vi "SNR.vi"(10 "ROI":T2, 11 "Refnum in":T1) -> (3 "SNR Results":T3)   [LabVIEW 2023]
uses:
  <vilib>/vision/Image Controls.llb/IMAQ Image.ctl
  <vilib>/vision/NI_Vision_Development_Module.lvlib
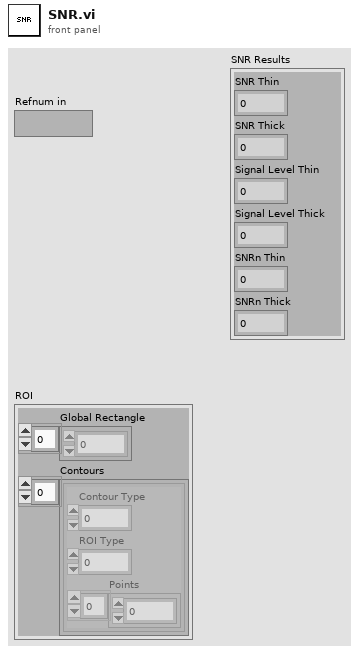
[diagram p1: front panel]
types:
  T1 = typedef "IMAQ Image.ctl" = refnum<image>
  T2 = cluster{"Global Rectangle":i32[], "Contours":cluster{"Contour Type":u32, "ROI Type":u32, "Points":i32[]}[]}
  T3 = cluster{"SNR Thin":sgl, "SNR Thick":sgl, "Signal Level Thin":sgl, "Signal Level Thick":sgl, "SNRn Thin":sgl, "SNRn Thick":sgl}
  T4 = typedef "ROI Descriptor" = cluster{"Global Rectangle":i32[], "Contours":cluster{"ID":enum32{"External", "Internal"}, "Type":u32, "Coordinates":i32[]}[]}
  T5 = cluster{"histogram":u32[], "Minimal Value":sgl, "Maximal Value":sgl, "Starting Value":sgl, "Interval Width":sgl, "Mean Value":sgl, "Standard  Variation":sgl, "Area (pixels)":i32}
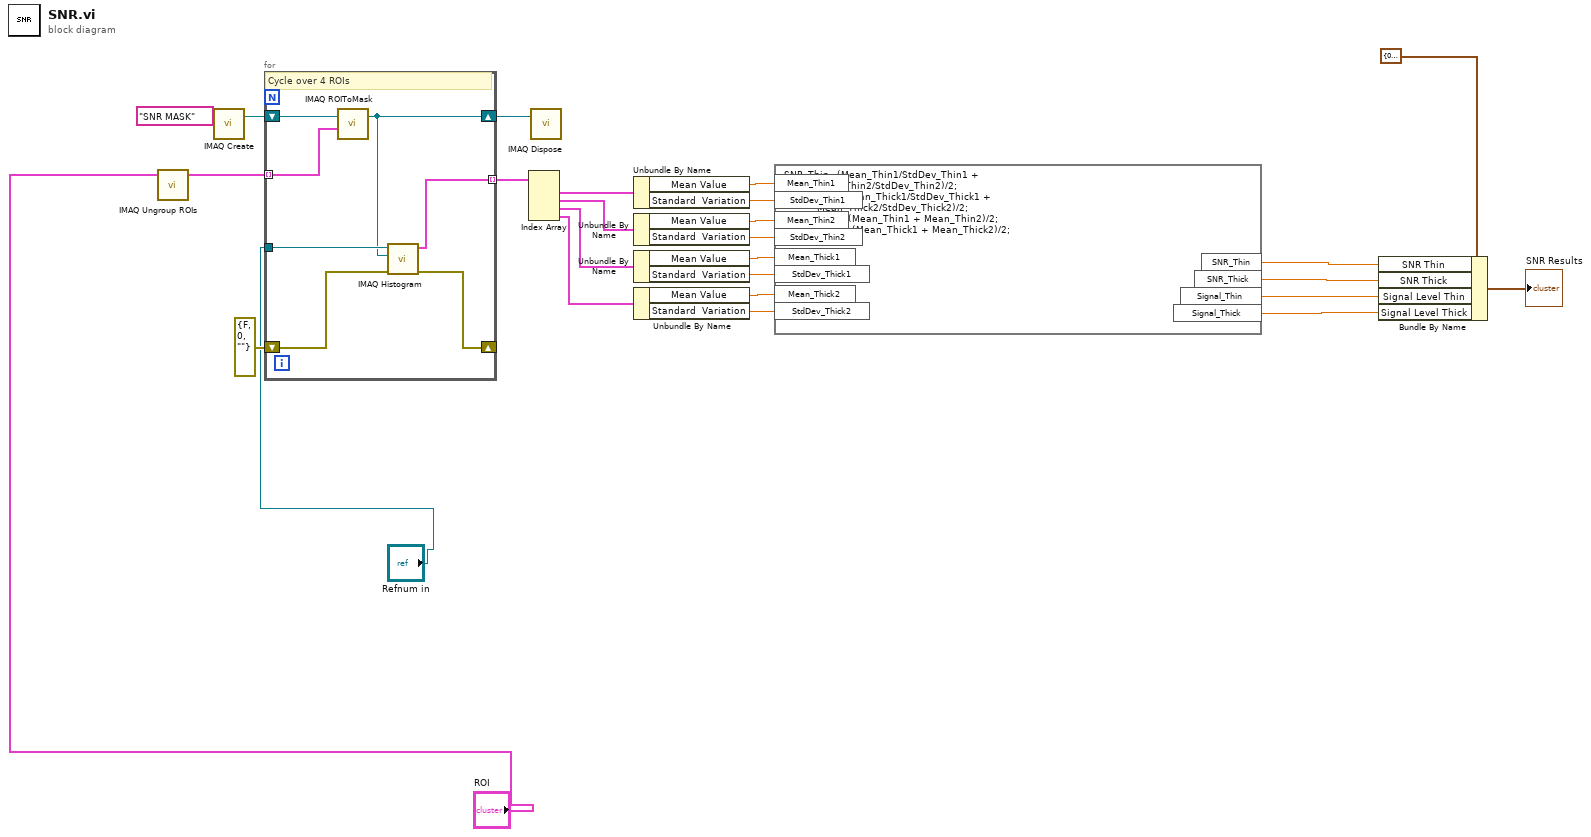
[diagram p0: block diagram]
diagram:
  n1 = call "IMAQ Ungroup ROIs"("ROI Descriptor"="ROI") -> ("ROI Descriptors out"=w3:T4[])  [unwired: 3 in, 1 out]
  n2 = call "IMAQ Create"("Image Name"="SNR MASK") -> ("New Image"=w5:T1)  [unwired: 3 in, 2 out]
  n3 = for {
    tunnel: "Refnum in" -> [w32]
    shift-right: [w28] -> _
    shift-left: errorcluster {"status"=FALSE, "code"=0, "source"=""} ("error out") -> [w31]
    tunnel: w3 -> [w30] mode=indexing
    shift-right: [w29] -> w2
    shift-left: w5 -> [w33]
    tunnel: [w27] -> w22 mode=indexing
    # "Cycle over 4 ROIs"
    n4 = call "IMAQ ROIToMask"("ROI Descriptor"=w30, "Image"=w33) -> ("Image Out"=w29:T1)  [unwired: 3 in, 3 out]
    n5 = call "IMAQ Histogram"("error in (no error)"=w31, "Image Mask"=w29, "Image"=w32) -> ("error out"=w28:errorcluster, "Histogram Report"=w27:T5)  [unwired: 2 in, 5 out]
  }
  n6 = Index Array(array=w22) -> (element #1=w6:T5, element #2=w7:T5, element #3=w8:T5, element #4=w9:T5)  [unwired: 4 in]
  n7 = call "IMAQ Dispose"("Image"=w2) -> ()  [unwired: 2 in, 4 out]
  n8 = Unbundle By Name(w6) -> ("Mean Value"=w10:sgl, "Standard  Variation"=w11:sgl)
  n9 = Unbundle By Name(w7) -> ("Mean Value"=w12:sgl, "Standard  Variation"=w13:sgl)
  n10 = Unbundle By Name(w8) -> ("Mean Value"=w14:sgl, "Standard  Variation"=w15:sgl)
  n11 = Unbundle By Name(w9) -> ("Mean Value"=w16:sgl, "Standard  Variation"=w17:sgl)
  n12 = formula code="SNR_Thin=(Mean_Thin1/StdDev_Thin1 + \n          Mean_Thin2/StdDev_Thin2)/2;\nSNR_Thick=(Mean_Thick1/StdDev_Thick1 + \n           Mean_Thick2/StdDev_Thick2)/2;\nSignal_Thin=(Mean_Thin1 + Mean_Thin2)/2;\nSignal_Thick=(Mean_Thick1 + Mean_Thick2)/2;"("Mean_Thin1"=w10, "Mean_Thin2"=w12, "StdDev_Thin1"=w11, "StdDev_Thin2"=w13, "Mean_Thick1"=w14, "StdDev_Thick1"=w15, "Mean_Thick2"=w16, "StdDev_Thick2"=w17) -> ("SNR_Thin"=w18:dbl, "SNR_Thick"=w19:dbl, "Signal_Thin"=w20:dbl, "Signal_Thick"=w21:dbl)
  n13 = Bundle By Name(cluster=T3 {"SNR Thin"=0.0, "SNR Thick"=0.0, "Signal Level Thin"=0.0, "Signal Level Thick"=0.0, "SNRn Thin"=0.0, "SNRn Thick"=0.0} ("SNR Results"), "SNR Thin"=w18, "SNR Thick"=w19, "Signal Level Thin"=w20, "Signal Level Thick"=w21) -> (→"SNR Results":T3)
